vi "保存数据.vi"(11 "账户信息":T1) -> (3 "账户信息 2":T1)   [LabVIEW 2018]
uses:
  <vilib>/Utility/file.llb/Read Delimited Spreadsheet (string).vi
  <vilib>/Utility/file.llb/Write Delimited Spreadsheet (string).vi
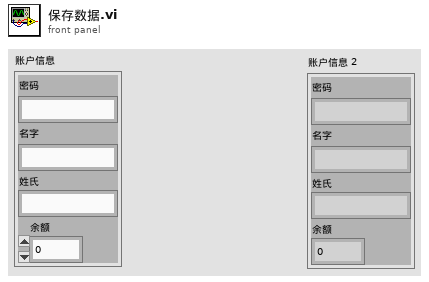
[diagram p1: front panel]
types:
  T1 = typedef "账户信息.ctl" = cluster{"密码":string, "名字":string, "姓氏":string, "余额":dbl}
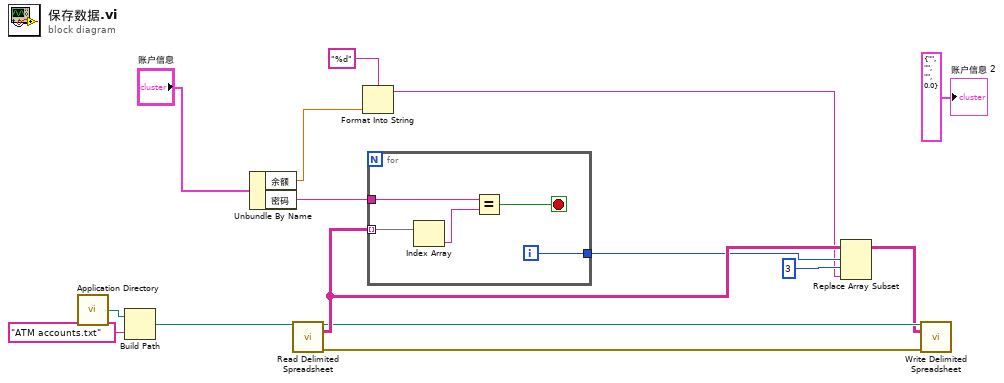
[diagram p0: block diagram]
diagram:
  n1 = call <vilib>:"Application Directory.vi"() -> ("Application Directory"=w15:path)
  n2 = Build Path(base path=w15, name or relative path="ATM accounts.txt" ("名称或相对路径")) -> (appended path=w13:path)
  n3 = Unbundle By Name("账户信息") -> ("余额"=w5:dbl, "密码"=w9:string)
  n4 = call-poly <vilib>:"Read Delimited Spreadsheet.vi"("file path (dialog if empty)"=w13) -> ("new file path (Not A Path if cancelled)"=w2:path, "all rows"=w8:string[][], "error out"=w12:errorcluster)  [unwired: 9 in, 3 out]
  n5 = Format Into String(format string="%d" ("格式字符串"), w5) -> (resulting string=w3:string)  [unwired: 2 in, 1 out]
  n6 = for {
    tunnel: w9 -> [w19]
    tunnel: w8 -> [w20] mode=indexing
    tunnel: [w16] -> w7
    i -> [w16]
    stop <- w17 stop-if-true
    n7 = Index Array(array=w20) -> (element=w18:string)  [unwired: 1 in]
    n8 = Equal?(x=w19, y=w18) -> (x = y?=w17:bool)
  }
  n9 = Replace Array Subset(array=w8, new element=w3, index (row)=w7, index (col)=3 ("禁用的索引 (列)")) -> (w1:string[][])
  n10 = call-poly <vilib>:"Write Delimited Spreadsheet.vi"("file path (dialog if empty)"=w2, "2D data"=w1, "error in (no error)"=w12) -> ()  [unwired: 11 in, 2 out]
  "账户信息 2" <- T1 {"密码"="", "名字"="", "姓氏"="", "余额"=0.0} ("账户信息 2")
